vi "CleanUp Diagram.vi"(8 "error in (no error)":errorcluster, 10 "Top Level Diagram":refnum<vi>, 11 "Initial Sequence in":refnum<class "Main Sequence.lvclass">) -> (0 "error out":errorcluster, 3 "Initial Sequence out":refnum<class "Main Sequence.lvclass">)   [LabVIEW 2015, in "Main Sequence.lvclass"]
uses:
  Main Sequence.lvclass
  Structures/Structures.lvclass/Structures.ctl
  Structures/Read Structure.vi
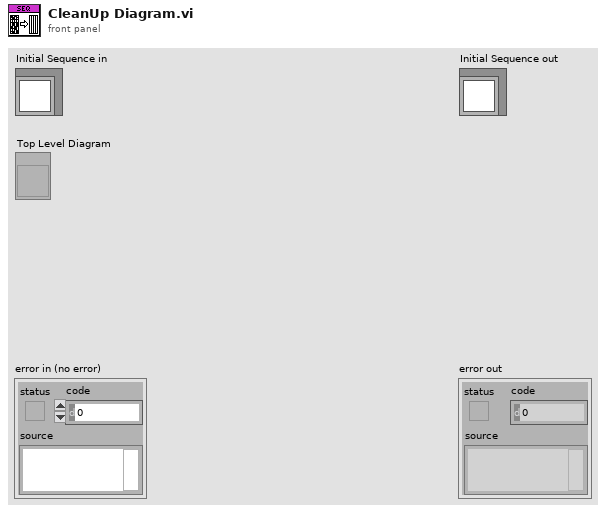
[diagram p1: front panel]
types:
  T1 = enum32{"Top Edges", "Vertical Centers", "Bottom Edges", "Left Edges", "Horizontal Centers", "Right Edges"}
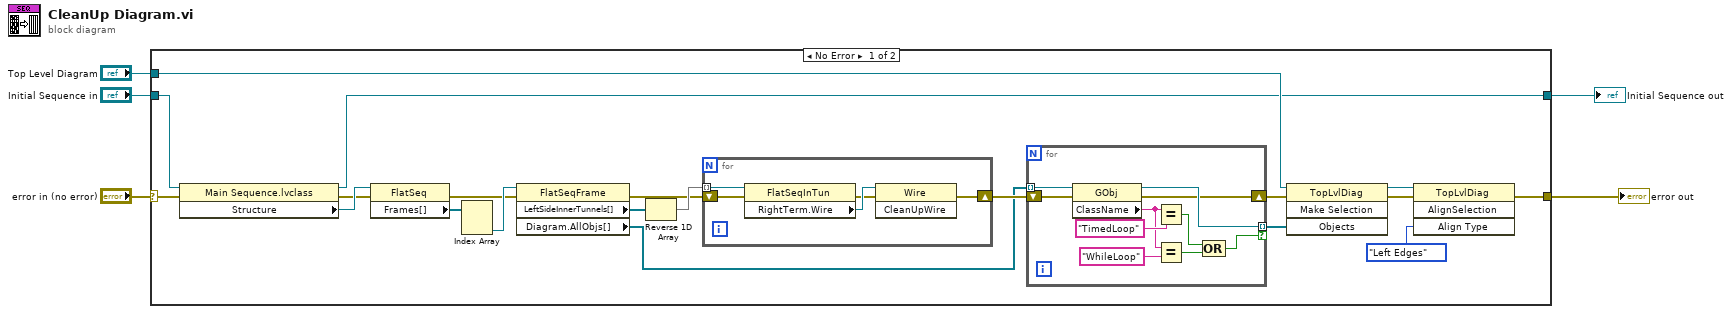
[diagram p0: block diagram]
diagram:
  n1 = case shown="No Error" "error in (no error)" {
    selector: "error in (no error)" -> [w13 w41]
    tunnel: "Initial Sequence in" -> [w14 w42]
    tunnel: "Top Level Diagram" -> [w12 _]
    tunnel: [w7 w41] -> w2
    tunnel: [w6 w42] -> w1
    frame No Error {
      n2 = property class="Main Sequence.lvclass"(reference=w14, error in=w13) -> (reference out=w6:refnum<class "Main Sequence.lvclass">, error out=w23:errorcluster, "Structure"=w25:refnum<vi>)
      n3 = property class="FlatSeq"(reference=w25, error in=w23) -> (error out=w18:errorcluster, "Frames[]"=w24:refnum<vi>[])  [unwired: 1 out]
      n4 = Index Array(array=w24) -> (element #2=w19:refnum<vi>)  [unwired: 2 in, 1 out]
      n5 = property class="FlatSeqFrame"(reference=w19, error in=w18) -> (error out=w8:errorcluster, "LeftSideInnerTunnels[]"=w16:refnum<vi>[], "Diagram.AllObjs[]"=w9:refnum<vi>[])  [unwired: 1 out]
      n6 = Reverse 1D Array(array=w16) -> (reversed array=w15:refnum<vi>[])
      n7 = for {
        tunnel: w15 -> [w30] mode=indexing
        shift-right: [w26] -> w10
        shift-left: w8 -> [w29]
        n8 = property class="FlatSeqInTun"(reference=w30, error in=w29) -> (error out=w27:errorcluster, "RightTerm.Wire"=w28:refnum<vi>)  [unwired: 1 out]
        n9 = invoke class="Wire" method="CleanUpWire"(reference=w28, error in=w27) -> (error out=w26:errorcluster)  [unwired: 1 in, 2 out]
      }
      n10 = for {
        tunnel: w9 -> [w40] mode=indexing
        tunnel: [w35] -> w17 mode=indexing if=w34
        shift-right: [w32] -> w11
        shift-left: w10 -> [w33]
        n11 = property class="GObj"(reference=w40, error in=w33) -> (reference out=w35:refnum<vi>, error out=w32:errorcluster, "ClassName"=w31:string)
        n12 = Equal?(x=w31, y="TimedLoop") -> (x = y?=w38:bool)
        n13 = Equal?(x=w31, y="WhileLoop") -> (x = y?=w36:bool)
        n14 = Compound Arithmetic op=OR(w38, w36) -> (w34:bool)
      }
      n15 = invoke class="TopLvlDiag" method="Make Selection"(reference=w12, error in=w11, "Objects"=w17) -> (reference out=w22:refnum<vi>, error out=w21:errorcluster)  [unwired: 1 in, 2 out]
      n16 = invoke class="TopLvlDiag" method="AlignSelection"(reference=w22, error in=w21, "Align Type"=T1."Left Edges") -> (error out=w7:errorcluster)  [unwired: 1 in, 3 out]
    }
    frame Error {
    }
  }
  "error out" <- w2
  "Initial Sequence out" <- w1
